vi "SourceOpenSynchronization.vi"(0 "error in (no error)":errorcluster, 5 "SourceData":cluster{"Tag":string, "Port":i32}[](array[cluster]), 6 "COM Port in":refnum<visa-resource-name>) -> (1 "Notifiers out":refnum<notifier>[](array[refnum]), 2 "Queue Reference out":refnum<notifier>[](array[refnum]), 3 "error out":errorcluster, 4 "Queue out":refnum<queue>, 9 "COM Port out":refnum<visa-resource-name>)   [LabVIEW 2009]
uses:
  Controls/SourceCommand.ctl
  Controls/SourceStatus.ctl
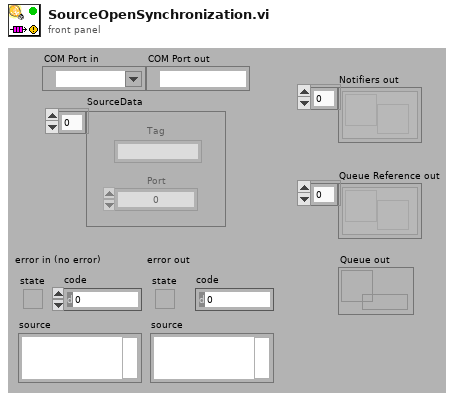
[diagram p1: front panel]
types:
  T1 = typedef "SourceCommand.ctl" = cluster{"Source":string, "Command":enum16{"INTENSITY", "ALL OFF", "QUIT"}, "Intensity":i32, "Ok?":refnum<k4>}
  T2 = typedef "SourceStatus.ctl" = cluster{"Managed?":bool, "Intensity":i32}
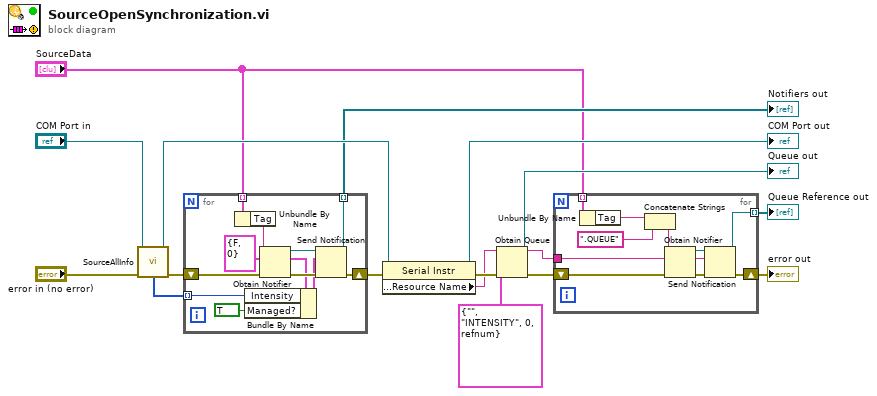
[diagram p0: block diagram]
diagram:
  n1 = call "SourceAllInfo.vi"("COM Port in"="COM Port in", "error in (no error)"="error in (no error)") -> ("COM Port out"=w9:refnum<visa-resource-name>, "error out"=w12:errorcluster, "Intensity"=w11:i32[])  [unwired: 5 out]
  n2 = for {
    shift-right: [w20] -> w10
    shift-left: w12 -> [w26]
    tunnel: [w24] -> w2 mode=indexing
    tunnel: "SourceData" -> [w16] mode=indexing
    tunnel: w11 -> [w22] mode=indexing
    w19 = T2 {"Managed?"=FALSE, "Intensity"=0} ("SourceStatus")
    n3 = Unbundle By Name(w16) -> ("Tag"=w17:string)
    n4 = Bundle By Name(cluster=w19, "Intensity"=w22, "Managed?"=TRUE) -> (w23:T2)
    n5 = Obtain Notifier(name (unnamed)=w17, notification data type=w19, error in (no error)=w26) -> (notifier out=w21:refnum<notifier>, error out=w25:errorcluster)  [unwired: 1 in, 1 out]
    n6 = Send Notification(notification=w23, notifier=w21, error in (no error)=w25) -> (notifier out=w24:refnum<notifier>, error out=w20:errorcluster)
  }
  "Notifiers out" <- w2
  n7 = property class="Serial Instr"(reference=w9, error in=w10) -> (reference out=→"COM Port out":refnum<visa-resource-name>, error out=w7:errorcluster, "General Settings:Resource Name"=w6:string)
  n8 = Obtain Queue(name (unnamed)=w6, element data type=T1 {"Source"="", "Command"=enum."INTENSITY", "Intensity"=0, "Ok?"=refnum} ("SourceCommand"), error in (no error)=w7) -> (queue out=→"Queue out":refnum<queue>, error out=→"error out":errorcluster)  [unwired: 2 in, 1 out]
  n9 = for {
    shift-right: [w32] -> _
    shift-left: _ -> [w36]
    tunnel: [w34] -> w5 mode=indexing
    tunnel: w6 -> [w29]
    tunnel: "SourceData" -> [w28] mode=indexing
    n10 = Unbundle By Name(w28) -> ("Tag"=w27:string)
    n11 = Concatenate Strings(w27, ".QUEUE") -> (w30:string)
    n12 = Obtain Notifier(name (unnamed)=w30, notification data type=w29, error in (no error)=w36) -> (notifier out=w33:refnum<notifier>, error out=w35:errorcluster)  [unwired: 1 in, 1 out]
    n13 = Send Notification(notification=w29, notifier=w33, error in (no error)=w35) -> (notifier out=w34:refnum<notifier>, error out=w32:errorcluster)
  }
  "Queue Reference out" <- w5
